vi "Global 1.vi"() -> ()   [LabVIEW 2019]
panel:
  out "negativo":dbl
  out "positivo":dbl
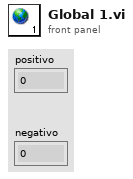
[diagram p1: front panel]
diagram:
